vi "Marvin.vi"() -> ()   [LabVIEW 2017]
uses:
  Fuse_LW/Fuse25A_Labview/CANalystII/PCAN_Driver/ControlCAN.llb/CAN Channel.ctl
  CAN TxRx/CAN/CANalystII/PCAN_Driver/ControlCAN.llb/DevType.ctl
  CAN TxRx/CAN/CANalystII/PCAN_Driver/ControlCAN.llb/VCI_INIT_CONFIG.ctl
  CAN TxRx/CAN/CANalystII/PCAN_Driver/ControlCAN.llb/InitFlag.ctl
  CAN TxRx/CAN/CANalystII/PCAN_Driver/ControlCAN.llb/Fliter.ctl
  CAN TxRx/CAN/CANalystII/PCAN_Driver/ControlCAN.llb/Mode.ctl
  CAN TxRx/CAN/CANalystII/PCAN_Driver/ControlCAN.lvlib
panel:
  in  "lock":bool=TRUE
  in  "Display":bool
  in  "address":u16=341 format="%.0x"
  out "UnitType":T1(ring)
  in  "ch2_old":dbl
  in  "ch1_old":dbl
  out "ADC Units 6":dbl
  out "Config_CANAT":T8 {"DevType" items=["USB-CAN"=3, "USB-CAN2"=4]; "CanIndex" items=["通道1", "通道2"]; "VCI_INIT_CONFIG"."Fliter" items=["接收所有类型"=3, "只接收标准帧"=4, "只接收扩展帧"=7]; "VCI_INIT_CONFIG"."Mode" items=["正常工作", "自测模式（环回）", "仅侦听模式"]; "VCI_INIT_CONFIG"."InitFlag" items=["使用Flash参数", "使用界面设置参数"]}
  in  "Channel 2":T3 caption="Channel" items=["Channel 1", "Channel 2"]
  in  "CANType":u16(ring) items=["LAWICEL", "PCAN", "CANalystII"]
  out "error out 7":errorcluster
  out "error out 2":errorcluster
  in  "Clear History":bool
  in  "Time":i32=-1
  out "History":string
  in  "Tab Control":T9(tab)
  in  "Status 1":bool
  in  "Status":bool
  in  "SN":string
  in  "Get Version":bool
  out "Unit PN":string
  out "SW ver":string
  in  "Get SN":bool
  in  "Set SN":bool
  in  "Get PN":bool
  in  "Clear Time Log":bool
  in  "Clear Log":bool
  out "Event Logs":string
  in  "Clear Event Logs":bool
  in  "TxID":u32 format="%.0x"
  in  "Data":u8[](array[numeric])
  in  "Sent Debug":bool
  in  "Unit SN":bool
  in  "Bootloader":bool
  in  "Ethernet Config. Data":string
  in  "SendData":bool
  in  "ReadParam":bool
  in  "Unit reset":bool
  in  "SW ver":bool
  in  "MAC address":bool
  out "RX Cnt":u32
  out "TX Cnt":u32
  in  "stop m":bool
  out "error out 5":errorcluster
  out "error out 6":errorcluster
  out "erroro5 2":errorcluster
  out "erroro5":errorcluster
  out "error out 4":errorcluster
  out "VISA res_out":refnum<visa-resource-name>
  in  "Seria- Port":refnum<visa-resource-name>="COM5"
  out "error out 3":errorcluster
  out "error02":errorcluster
  out "error out":errorcluster
  out "RX":bool
  out "TX":bool
  in  "Disonnect":bool
  in  "Connect":bool
  out "CommIcon":bool=TRUE
  in  "UIFlagStop":bool
  in  "RXFlagStop":bool
  in  "TXFlagStop":bool
  out "Error":string
  out "Adapter Version":string
  in  "Baud":u16(ring)=284 items=["1M"=20, "500K"=28, "250K"=284, "125K"=796, "100K"=17199, "50K"=18223, "20K"=21295, "10K"=26415, "5K"=32639]
  # "[msec]"
  # "Save Data"
  # "[sec]"
  # "[msec]"
  # "DO 3"
  # "DO 4"
  # "DO 5"
  # "DO 6"
  # "DO 7"
  # "DO 8"
  # "DO 9"
  # "DO 10"
  # "DO 11"
  # "DO 12"
  # "DO 13"
  # "DO 14"
  # "DO 15"
  # "DO 16"
  # "ver 1.0"
  # "Channel Parameter"
  # "** 0-Infinity"
  # "System Parameters"
  # "Digital input status"
  # "*255-Infinity"
  # "DI 17"
  # "DI 18"
  # "DI 19"
  # "**"
  # "DI 20"
  # "DI 21"
  # "DI 22"
  # "DI 23"
  # "DI 24"
  # "DI 25"
  # "*"
  # "DI 26"
  # "DI 27"
  # "DI 28"
  # "*65535-always On"
  # "*"
  # "*65535-OFF"
  # "OC command"
  # "OC1"
  # "BIT"
  # "Production Data"
  # "OC2"
  # "Unit S/N"
  # "Offset Data"
  # "Custom Message"
  # "Channel Data"
  # "Channel Protection"
  # "Marvin"
  # "REDLER TECHNOLOGIES LTD"
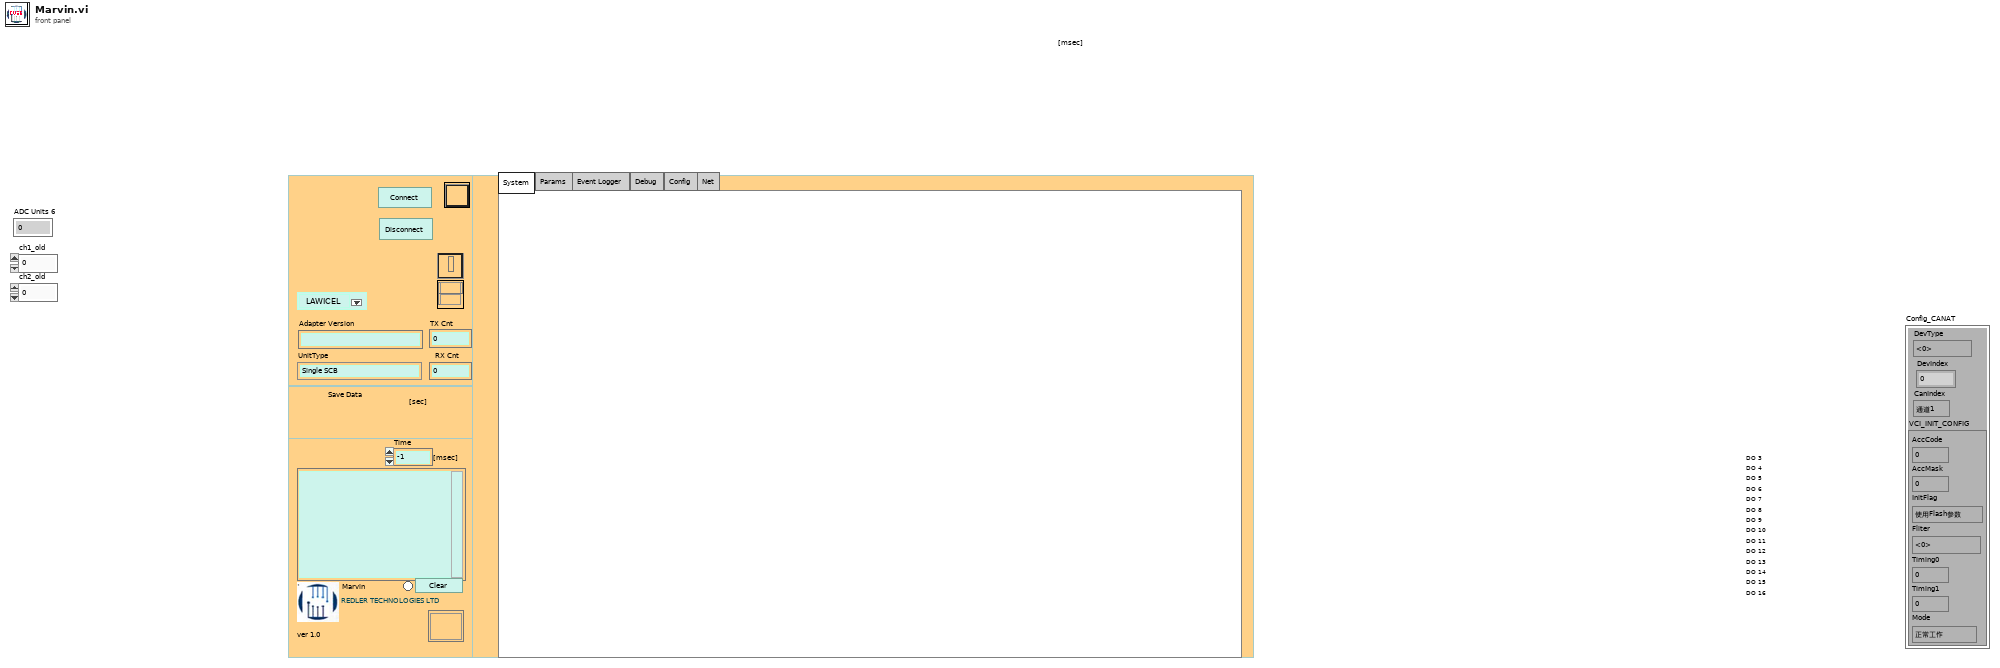
[diagram p1: front panel]
types:
  T1 = enum16{"Single SCB", "Power Rider", "Power Rider&Next10", "HATAL", "DAPH", "Indefinite", "Power Rider 12"}
  T2 = typedef "ControlCAN.lvlib/DevType.ctl" = u32
  T3 = typedef "ControlCAN.lvlib/CAN Channel.ctl" = u32
  T4 = typedef "ControlCAN.lvlib/VCI_INIT_CONFIG.ctl" = cluster{"AccCode":u32, "AccMask":u32, "InitFlag":T5, "Fliter":T6, "Timing0":u8, "Timing1":u8, "Mode":T7}
  T5 = typedef "ControlCAN.lvlib/InitFlag.ctl" = u32
  T6 = typedef "ControlCAN.lvlib/Fliter.ctl" = u8
  T7 = typedef "ControlCAN.lvlib/Mode.ctl" = u8
  T8 = cluster{"DevType":T2, "DevIndex":u32, "CanIndex":T3, "VCI_INIT_CONFIG":T4}
  T9 = enum32{"System", "Params", "Event Logger", "Debug", "Config", "Net"}
  T10 = enum16{"Single SCB", "Power Rider", "Power Rider&Next10", "HATAL", "DAPH", "Indefinite"}
  T11 = cluster{"ID":u32, "MSGTYPE":u8, "LEN":u8, "aDATA":u8[]}
  T12 = typedef "PCAN_ERROR.ctl" = i32
  T13 = cluster{"Is Warning":bool, "Is Error":bool, "Message":string}
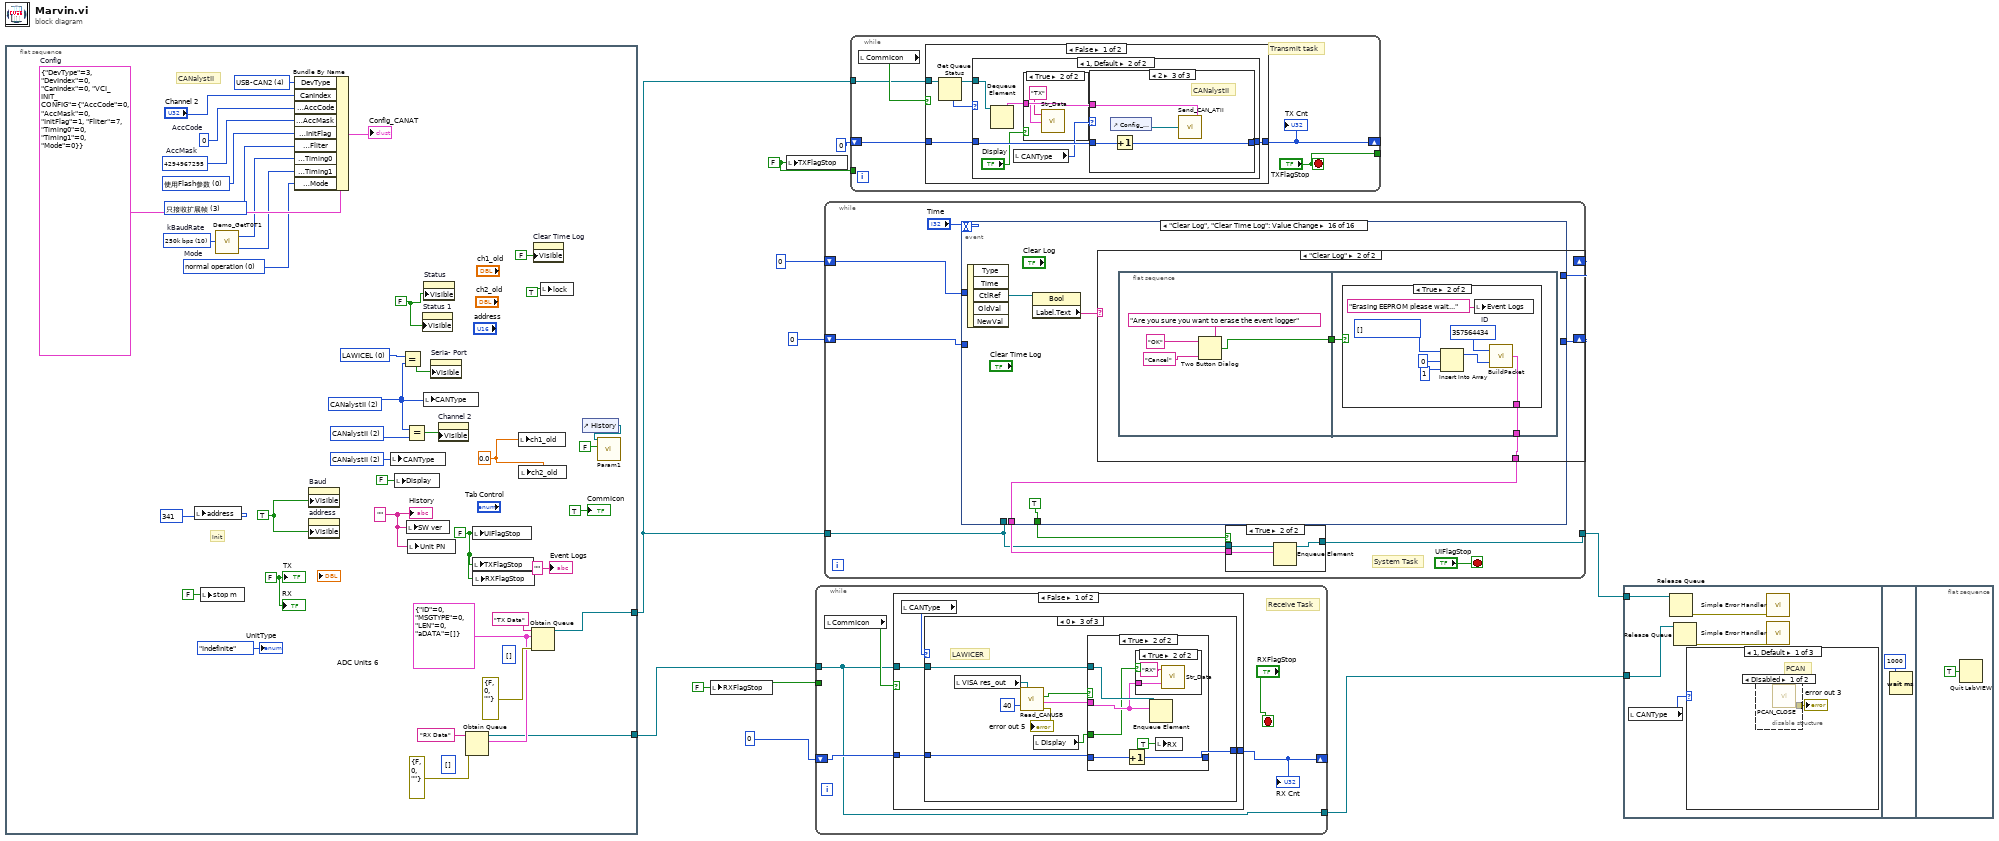
[diagram p0: block diagram]
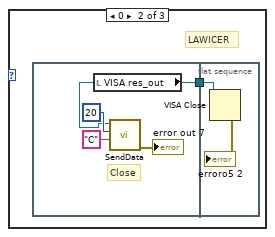
[diagram p3: hidden frame]
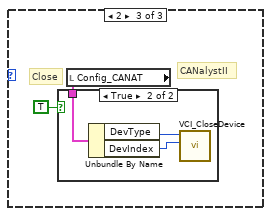
[diagram p4: hidden frame]
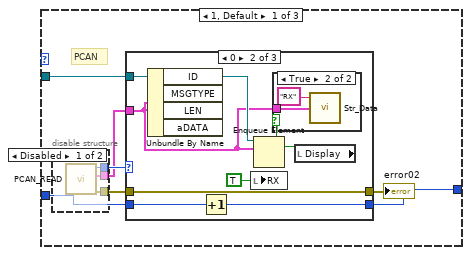
[diagram p6: hidden frame]
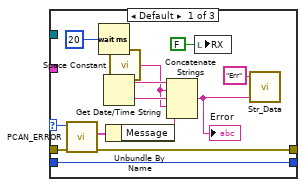
[diagram p8: hidden frame]
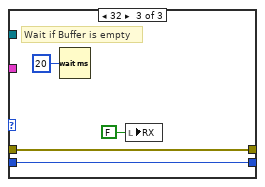
[diagram p10: hidden frame]
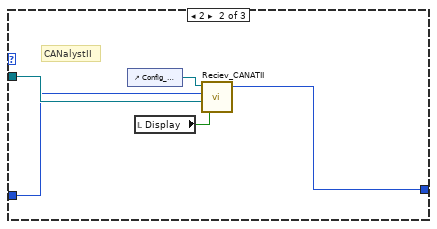
[diagram p11: hidden frame]
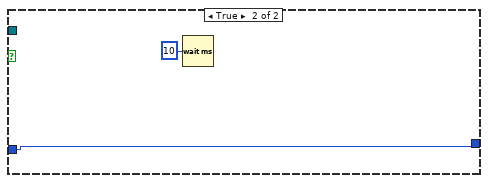
[diagram p14: hidden frame]
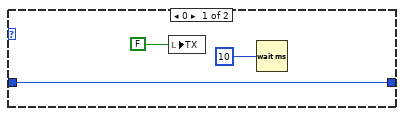
[diagram p15: hidden frame]
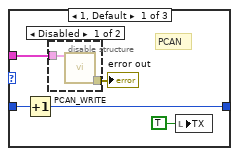
[diagram p17: hidden frame]
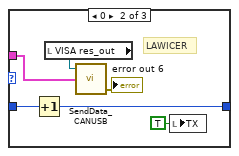
[diagram p19: hidden frame]
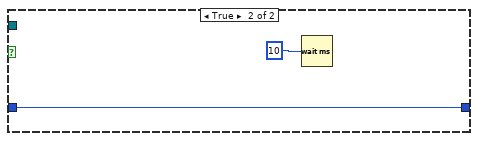
[diagram p20: hidden frame]
diagram:
  w4 = FALSE ("TXFlagStop")
  w5 = FALSE ("RXFlagStop")
  n1 = flat-sequence {
    tunnel: [w47] -> w8
    tunnel: [w45] -> w7
    frame #0 {
      w17 = "" ("str out")
      w19 = 0.0 ("ch1_old")
      w26 = TRUE ("Visible")
      w25 = u16 2 items=["LAWICEL", "PCAN", "CANalystII", "TCP Client", "TCP Server"] ("CANType")
      w23 = u16 2 items=["LAWICEL", "PCAN", "CANalystII", "TCP Client", "TCP Server"] ("CANType")
      w24 = u16 2 items=["LAWICEL", "PCAN", "CANalystII", "TCP Client", "TCP Server"] ("CANType")
      w22 = u16 0 items=["LAWICEL", "PCAN", "CANalystII", "TCP Client", "TCP Server"] ("CANType")
      w39 = u32 4294967295  # AccMask
      w38 = T5 0 items=["使用Flash参数", "使用界面设置参数"] ("InitFlag")
      w33 = T7 0 items=["normal operation", "Listen-only mode", "test mode"]  # Mode
      w37 = T6 3 items=["接收所有类型"=1, "只接收标准帧"=2, "只接收扩展帧"=3] ("Fliter")
      w36 = u8 10 items=["5k bps"=1, "10k bps"=2, "20k bps"=3, "40k bps"=4, "50k bps"=5, "80k bps"=6, "100k bps"=7, "125k bps"=8, "200k bps"=9, "250k bps"=10, "400k bps"=11, "500k bps"=12, "666k bps"=13, "800k bps"=14, "1000k bps"=15, "33.33k bps"=16, "66.66k bps"=17, "83.33k bps"=18]  # kBaudRate
      w40 = u32 0  # AccCode
      w42 = T2 4 items=["USB-CAN"=3, "USB-CAN2"=4] ("DevType")
      w43 = T8 {"DevType"=3, "DevIndex"=0, "CanIndex"=0, "VCI_INIT_CONFIG"={"AccCode"=0, "AccMask"=0, "InitFlag"=1, "Fliter"=7, "Timing0"=0, "Timing1"=0, "Mode"=0}}  # Config
      w31 = FALSE ("Visible")
      w27 = FALSE ("TX")
      w46 = T11 {"ID"=0, "MSGTYPE"=0, "LEN"=0, "aDATA"=[]} ("Msg")
      (unwired) u8[] []
      (unwired) u8[] []
      w11 = FALSE ("UIFlagStop")
      # "CANalystII"
      # "Init"
      n2 = local write "address"(u16 341 ("address-type")) -> ()
      n3 = local write "stop m"(FALSE ("stop m")) -> ()
      n4 = call "Demo_GetT0T1.vi"("kBaudRate"=w36) -> ("Timing0"=w35:u8, "Timing1"=w34:u8)
      n5 = Bundle By Name(cluster=w43, "DevType"=w42, "CanIndex"="Channel 2", "VCI_INIT_CONFIG.AccCode"=w40, "VCI_INIT_CONFIG.AccMask"=w39, "VCI_INIT_CONFIG.InitFlag"=w38, "VCI_INIT_CONFIG.Fliter"=w37, "VCI_INIT_CONFIG.Timing0"=w35, "VCI_INIT_CONFIG.Timing1"=w34, "VCI_INIT_CONFIG.Mode"=w33) -> (→"Config_CANAT":T8)
      n6 = property on="Baud" class="Ring (strict)"("Visible"=w26) -> ()  [unwired: 2 in, 2 out]
      n7 = property on="address" class="DigNum (strict)"("Visible"=w26) -> ()  [unwired: 2 in, 2 out]
      n8 = local write "CANType"(w25) -> ()
      n9 = local write "Display"(FALSE ("Display")) -> ()
      n10 = Equal?(x=w22, y=w24) -> (x = y?=w20:bool)
      n11 = Equal?(x=w24, y=w23) -> (x = y?=w21:bool)
      n12 = local write "SW ver"(w17) -> ()
      n13 = local write "Unit PN"(w17) -> ()
      n14 = property on="Status 1" class="Bool"("Visible"=w31) -> ()  [unwired: 2 in, 2 out]
      n15 = local write "CANType"(w24) -> ()
      n16 = property on="Status" class="Bool"("Visible"=w31) -> ()  [unwired: 2 in, 2 out]
      n17 = property on="Seria- Port" class="VISAName"("Visible"=w20) -> ()  [unwired: 2 in, 2 out]
      n18 = property on="Channel 2" class="Ring (strict)"("Visible"=w21) -> ()  [unwired: 2 in, 2 out]
      n19 = Obtain Queue(name (unnamed)="RX Data", element data type=w46, error in (no error)=errorcluster {"status"=FALSE, "code"=0, "source"=""}) -> (queue out=w45:refnum<queue>)  [unwired: 2 in, 2 out]
      n20 = local write "UIFlagStop"(w11) -> ()
      n21 = local write "TXFlagStop"(w11) -> ()
      n22 = local write "RXFlagStop"(w11) -> ()
      n23 = local write "ch1_old"(w19) -> ()
      n24 = local write "ch2_old"(w19) -> ()
      n25 = Obtain Queue(name (unnamed)="TX Data", element data type=w46, error in (no error)=errorcluster {"status"=FALSE, "code"=0, "source"=""}) -> (queue out=w47:refnum<queue>)  [unwired: 2 in, 2 out]
      n26 = property on="Clear Time Log" class="Bool"("Visible"=FALSE) -> ()  [unwired: 2 in, 2 out]
      n27 = local write "lock"(TRUE ("lock")) -> ()
      n28 = control-ref of="History"() -> (w16:refnum<vi>)
      n29 = call "Param1.vi"("str"=w16, "Init_F"=FALSE) -> ()  [unwired: 16 in, 2 out]
      "RX" <- w27
      "TX" <- w27
      "Event Logs" <- "" ("Event Logs")
      "UnitType" <- T10."Indefinite" ("UnitType")
      "CommIcon" <- TRUE ("CommIcon")
      "History" <- w17
    }
  }
  n30 = local write "RXFlagStop"(w5) -> ()
  n31 = local write "TXFlagStop"(w4) -> ()
  n32 = while {
    tunnel: w7 -> [w52]
    shift-right: [w53] -> _
    shift-left: u32 0 ("cnt_out") -> [w54]
    tunnel: w5 -> [_]
    tunnel: [w52] -> w2
    stop <- "RXFlagStop" stop-if-true
    # "Receive Task"
    n33 = local read "CommIcon"() -> (w55:bool)
    n34 = case shown="False" w55 {
      tunnel: w52 -> [w60 _]
      tunnel: w54 -> [w58 w120]
      tunnel: [w57 w120] -> w53
      frame False {
        n35 = local read "CANType"() -> (w59:u16)
        n36 = case shown="0" w59 {
          tunnel: w60 -> [w64 w100 w107]
          tunnel: w58 -> [w62 w99 w104]
          tunnel: [w61 w98 w103] -> w57
          frame 1, Default {
            # "PCAN"
            n37 = disable-structure shown="Disabled" {
              disable-tunnel: [w70 _] -> w67
              disable-tunnel: [w69 _] -> w66
              disable-tunnel: [w68 _] -> w65
              frame Disabled {
                n38 = call "PCAN_READ.vi"() -> ("error out"=w70:errorcluster, "TPCANMsg"=w68:T11, "error"=w69:T12)  [unwired: 2 in, 7 out]
              }
              frame Enabled {
              }
            }
            n39 = case shown="0" w66 {
              selector: w66 -> [w82 _ _]
              tunnel: w65 -> [_ w86 _]
              tunnel: w67 -> [w83 w90 w95]
              tunnel: [w81 w90 w95] -> w63
              tunnel: w64 -> [_ w89 _]
              tunnel: w62 -> [w73 w85 w93]
              tunnel: [w73 w87 w93] -> w61
              frame Default {
                n40 = call "PCAN_ERROR.vi"("error in (no error)"=w83, "Error Code"=w82) -> ("error out"=w81:errorcluster, "PCAN error"=w80:T13)  [unwired: 8 out]
                n41 = Wait (ms)(milliseconds to wait=u32 20) -> ()  [unwired: 1 out]
                n42 = Get Date/Time String() -> (date string=w78:string, time string=w77:string)  [unwired: 3 out]
                n43 = Unbundle By Name(w80) -> ("Message"=w76:string)
                n44 = call <vilib>:"Space Constant.vi"() -> ("String"=w75:string)
                n45 = Concatenate Strings(w78, w75, w77, w75, w76) -> (w71:string)
                "Error" <- w71
                n46 = local write "RX"(FALSE ("RX")) -> ()
                n47 = call "Str_Data.vi"("Err str"=w71, "string"="Err") -> ()  [unwired: 1 in, 1 out]
              }
              frame 0 {
                n48 = Unbundle By Name(w86) -> ()  [unwired: 4 out]
                n49 = Increment(x=w85) -> (x+1=w87:u32)
                n50 = local write "RX"(TRUE ("RX")) -> ()
                n51 = Enqueue Element(queue=w89, element=w86) -> ()  [unwired: 1 in, 4 out]
                n52 = local read "Display"() -> (w84:bool)
                n53 = case shown="True" w84 {
                  tunnel: w86 -> [_ w91]
                  frame False {
                  }
                  frame True {
                    n54 = call "Str_Data.vi"("Msg"=w91, "string"="RX") -> ()  [unwired: 1 in, 1 out]
                  }
                }
              }
              frame 32 {
                # "Wait if Buffer is empty"
                n55 = Wait (ms)(milliseconds to wait=u32 20) -> ()  [unwired: 1 out]
                n56 = local write "RX"(FALSE ("RX")) -> ()
              }
            }
            "error02" <- w63
          }
          frame 2 {
            # "CANalystII"
            n57 = control-ref of="Config_CANAT"() -> (w101:refnum<vi>)
            n58 = local read "Display"() -> (w97:bool)
            n59 = call "Reciev_CANATII.vi"("Display"=w97, "queue out"=w100, "cnd_in"=w99, "Config"=w101) -> ("cnt_out"=w98:u32)  [unwired: 2 out]
          }
          frame 0 {
            # "LAWICER"
            n60 = local read "VISA res_out"() -> (w110:refnum<visa-resource-name>)
            n61 = call "Read_CANUSB.vi"("VISA  in"=w110, "byte count"=u32 40) -> ("Status"=w105:bool, "TPCANMsg out"=w106:T11, "error out 5"=→"error out 5":errorcluster)  [unwired: 2 out]
            n62 = local read "Display"() -> (w102:bool)
            n63 = case shown="True" w105 {
              tunnel: w107 -> [_ w116]
              tunnel: w106 -> [_ w113]
              tunnel: w104 -> [w111 w115]
              tunnel: [w111 w114] -> w103
              tunnel: w102 -> [_ w112]
              frame False {
              }
              frame True {
                n64 = Increment(x=w115) -> (x+1=w114:u32)
                n65 = case shown="True" w112 {
                  tunnel: w113 -> [_ w118]
                  frame False {
                  }
                  frame True {
                    n66 = call "Str_Data.vi"("Msg"=w118, "string"="RX") -> ()  [unwired: 1 in, 1 out]
                  }
                }
                n67 = Enqueue Element(queue=w116, element=w113) -> ()  [unwired: 1 in, 4 out]
                n68 = local write "RX"(TRUE ("RX")) -> ()
              }
            }
          }
        }
      }
      frame True {
        n69 = Wait (ms)(milliseconds to wait=u32 10) -> ()  [unwired: 1 out]
      }
    }
    "RX Cnt" <- w53
  }
  n70 = while {
    tunnel: w8 -> [w128]
    tunnel: [w127] -> w1
    shift-right: [w125] -> _
    shift-left: u32 0 -> [w126]
    shift-right: [w123] -> _
    shift-left: u32 0 -> [w124]
    stop <- "UIFlagStop" stop-if-true
    # "System Task"
    n71 = event shown="[15] \"Clear Log\", \"Clear Time Log\": Value Change" {
      selector: _ -> [_ _ _ _ _ _ _ _ _ _ _ _ _ _ _ _]
      dyn-events: _ -> [_ _ _ _ _ _ _ _ _ _ _ _ _ _ _ _]
      timeout: "Time" -> [_ _ _ _ _ _ _ _ _ _ _ _ _ _ _ _]
      tunnel: [_ w141 _ w164 _ w206 w212 w218 _ _ w251 w253 _ _ _ w283] -> w131
      tunnel: [_ TRUE ("TX") FALSE ("TX") w165 FALSE TRUE TRUE TRUE FALSE FALSE TRUE _ FALSE FALSE _ TRUE] -> w130
      tunnel: w126 -> [_ _ w159 _ _ _ _ _ _ w237 _ _ _ _ _ _]
      tunnel: [_ _ w159 _ _ _ _ _ _ w237 _ _ _ _ _ _] -> w125
      tunnel: w128 -> [_ _ _ _ _ _ _ _ _ _ _ _ _ _ _ _]
      tunnel: w124 -> [_ _ w160 _ _ _ w208 w214 w220 _ w248 _ _ _ _ _]
      tunnel: [_ _ w160 _ _ _ w208 w214 w220 _ w248 _ _ _ _ _] -> w123
      event Timeout {
        n72 = event-data() -> ()  [unwired: 1 in, 1 out]
      }
      event "SendData", "ReadParam", "Unit reset", "SW ver", "Bootloader", "Unit SN", "MAC address": Value Change {
        w146 = u8 2 items=["STATUS"=128, "EXTENDED"=2, "RTR"=1, "DATA MSG"=0] ("MSGTYPE")
        n73 = event-data() -> ("CtlRef"=w139:refnum<vi>)  [unwired: 1 in]
        n74 = property class="Bool"(reference=w139) -> ("Label.Text"=w138:string)  [unwired: 1 in, 2 out]
        n75 = case shown="\"SendData\"" w138 {
          tunnel: ["" ("Ethernet Configuration Data") "Ethernet Config. Data" "netparam" ("Ethernet Configuration Data") "reset" ("Ethernet Configuration Data") "version" ("Ethernet Configuration Data") "boot" ("Ethernet Configuration Data") "serial" ("Ethernet Configuration Data") "mac" ("Ethernet Configuration Data")] -> w137
          frame "False", Default {
          }
          frame "SendData" {
          }
          frame "ReadParam" {
            # "read param."
          }
          frame "Unit reset" {
            # "reset"
          }
          frame "SW ver" {
            # "sw ver"
          }
          frame "Bootloader" {
            # "Bootloader"
          }
          frame "Unit SN" {
            # "S/N"
          }
          frame "MAC address" {
            # "MAC"
          }
        }
        n76 = String To Byte Array(string=w137) -> (unsigned byte array=w136:u8[])
        n77 = Array Size(array=w136) -> (size(s)=w143:i32)
        n78 = To Unsigned Byte Integer(number=w143) -> (unsigned 8bit integer=w145:u8)
        n79 = Bundle By Name(cluster=T11 {"ID"=0, "MSGTYPE"=0, "LEN"=0, "aDATA"=[]} ("MsgTX 2"), "ID"=u32 0, "MSGTYPE"=w146, "LEN"=w145, "aDATA"=w136) -> (w141:T11)
      }
      event "lock": Value Change {
        n80 = event-data() -> ()  [unwired: 1 in, 1 out]
        n81 = call "EnterPW.vi"() -> ("Prod"=w155:bool, "Tech"=w158:bool)  [unwired: 7 in, 2 out]
        n82 = Or(x=w158, y=w155) -> (x .or. y?=w157:bool)
        n83 = Not(x=w157) -> (.not. x?=w156:bool)
        n84 = call "PWVisibleCntl.vi"("Tech"=w158, "Product"=w155) -> ()  [unwired: 14 in]
        n85 = local write "lock"(w156) -> ()
        n86 = property on="Clear Time Log" class="Bool"("Visible"=w155) -> ()  [unwired: 2 in, 2 out]
      }
      event "Connect": Value Change {
        w167 = 0 items=["extended", "standart"] ("type")
        n87 = event-data() -> ()  [unwired: 1 in, 1 out]
        n88 = case shown="2" "CANType" {
          tunnel: [w178 w186 w197] -> w163
          tunnel: [w180 "CANalystII" ("read ver") w198] -> w166
          tunnel: "Baud" -> [w177 w189 w196]
          tunnel: w167 -> [w176 w188 _]
          frame 1, Default {
            # "PCAN"
            n89 = disable-structure shown="Disabled" {
              disable-tunnel: [w184 _] -> w180
              disable-tunnel: [w183 _] -> w179
              disable-tunnel: w177 -> [w182 _]
              disable-tunnel: w176 -> [w181 _]
              frame Disabled {
                n90 = call "Init_PCAN.vi"("type"=w181, "baud"=w182) -> ("Boolean"=w183:bool, "Version"=w184:string)
              }
              frame Enabled {
              }
            }
            n91 = Not(x=w179) -> (.not. x?=w178:bool)
          }
          frame 2 {
            # "CANalystII"
            n92 = flat-sequence {
              tunnel: w189 -> [w192]
              tunnel: w188 -> [_]
              tunnel: [w191] -> w185
              tunnel: [w194] -> w187
              tunnel: w185 -> [w193]
              frame #0 {
                n93 = control-ref of="Config_CANAT"() -> (w191:refnum<vi>)
                n94 = call "ChangeCANBaud.vi"("baud in"=w192, "reference"=w191) -> ()
              }
              frame #1 {
                n95 = call "InitCAN_ATII.vi"("Config"=w193) -> ("Sts"=w194:bool)
              }
            }
            n96 = Not(x=w187) -> (.not. x?=w186:bool)
          }
          frame 0 {
            # "LAWICER"
            n97 = call "Init_Lawicel.vi"("baud"=w196, "Seria- Port"="Seria- Port") -> ("error out 4"=→"error out 4":errorcluster, "Status"=w195:bool, "read ver"=w198:string, "VISA res_out"=→"VISA res_out":refnum<visa-resource-name>)  [unwired: 1 in]
            n98 = Not(x=w195) -> (.not. x?=w197:bool)
          }
        }
        "Adapter Version" <- w166
        n99 = Not(x=w163) -> (.not. x?=w162:bool)
        n100 = case shown="True" w162 {
          tunnel: [FALSE TRUE] -> w165
          tunnel: [T11 {"ID"=0, "MSGTYPE"=0, "LEN"=0, "aDATA"=[]} ("MsgTX 2") w172] -> w164
          frame False {
          }
          frame True {
            w174 = u32 357564455  # ID
            # "PN"
            # "0x15500027"
            n101 = call "BuildPacket.vi"("Data"=u8[] [] ("Data 2"), "TxID"=w174) -> ("MsgTX 2"=w172:T11)
          }
        }
        n102 = local write "CommIcon"(w163) -> ()
      }
      event "stop m": Value Change {
        w202 = TRUE ("UIFlagStop")
        n103 = event-data() -> ()  [unwired: 1 in, 1 out]
        n104 = local write "UIFlagStop"(w202) -> ()
        n105 = local write "TXFlagStop"(w202) -> ()
        n106 = local write "RXFlagStop"(w202) -> ()
      }
      event "Sent Debug": Value Change {
        n107 = event-data() -> ()  [unwired: 1 in, 1 out]
        n108 = call "BuildPacket.vi"("Data"="Data", "TxID"="TxID") -> ("MsgTX 2"=w206:T11)
      }
      event "Get Version": Value Change {
        w210 = u32 357564425  # ID
        # "Version"
        # "0x15500009"
        n109 = event-data() -> ()  [unwired: 1 in, 1 out]
        n110 = call "BuildPacket.vi"("Data"=u8[] [] ("Data 2"), "TxID"=w210) -> ("MsgTX 2"=w212:T11)
        "SW ver" <- "" ("SW ver")
      }
      event "Get PN": Value Change {
        w216 = u32 357564455  # ID
        # "P/N"
        # "0x15500027"
        n111 = event-data() -> ()  [unwired: 1 in, 1 out]
        n112 = call "BuildPacket.vi"("Data"=u8[] [] ("Data 2"), "TxID"=w216) -> ("MsgTX 2"=w218:T11)
        "Unit PN" <- "" ("SW ver")
      }
      event "Get SN", "Set SN": Value Change {
        # "SN"
        n113 = event-data() -> ("CtlRef"=w222:refnum<vi>)  [unwired: 1 in]
        n114 = property class="Bool"(reference=w222) -> ("Label.Text"=w221:string)  [unwired: 1 in, 2 out]
        n115 = case shown="\"Get SN\", Default" w221 {
          frame "Get SN", Default {
            n116 = call "SN_Data.vi"("type"=1) -> ()  [unwired: 10 in, 1 out]
            n117 = local write "SN"("" ("SN")) -> ()
          }
          frame "Set SN" {
            n118 = call "SN_Data.vi"("type"=0, "String"="SN") -> ()  [unwired: 9 in, 1 out]
          }
        }
      }
      event "CANType": Value Change {
        w234 = u16 2 items=["LAWICEL", "PCAN", "CANalystII"] ("CANType")
        w235 = u16 0 items=["LAWICEL", "PCAN", "CANalystII"] ("CANType")
        n119 = event-data() -> ()  [unwired: 1 in, 1 out]
        n120 = local read "CANType"() -> (w231:u16)
        n121 = case shown="1" w231 {
          tunnel: [w241 w244 w247] -> w230
          tunnel: [w241 w244 w247] -> w229
          tunnel: [FALSE ("TX") FALSE ("TX") FALSE ("TX")] -> _
          tunnel: [FALSE ("TX") FALSE ("TX") FALSE ("TX")] -> w228
          frame 0, Default {
            w241 = TRUE ("TX")
            # "Lawicel"
          }
          frame 1 {
            w244 = TRUE ("TX")
            # "PCAN"
          }
          frame 2 {
            w247 = TRUE ("TX")
            # "CANalystll"
          }
        }
        n122 = property on="Connect" class="Bool"("Visible"=w229) -> ()  [unwired: 2 in, 2 out]
        n123 = property on="Disonnect" class="Bool"("Visible"=w229) -> ()  [unwired: 2 in, 2 out]
        n124 = property on="Baud" class="Ring (strict)"("Visible"=w230) -> ()  [unwired: 2 in, 2 out]
        n125 = property on="address" class="DigNum (strict)"("Visible"=w230) -> ()  [unwired: 2 in, 2 out]
        n126 = local read "CANType"() -> (w232:u16)
        n127 = Equal?(x=w235, y=w232) -> (x = y?=w236:bool)
        n128 = Equal?(x=w232, y=w234) -> (x = y?=w233:bool)
        n129 = local write "CANType"(w232) -> ()
        n130 = property on="Channel 2" class="Ring (strict)"("Visible"=w233) -> ()  [unwired: 2 in, 2 out]
        n131 = property on="Seria- Port" class="VISAName"("Visible"=w236) -> ()  [unwired: 2 in, 2 out]
        n132 = property on="SendData" class="Bool"("Visible"=w228) -> ()  [unwired: 2 in, 2 out]
        n133 = property on="ReadParam" class="Bool"("Visible"=w228) -> ()  [unwired: 2 in, 2 out]
        n134 = property on="Unit reset" class="Bool"("Visible"=w228) -> ()  [unwired: 2 in, 2 out]
        n135 = property on="SW ver" class="Bool"("Visible"=w228) -> ()  [unwired: 2 in, 2 out]
        n136 = property on="Unit SN" class="Bool"("Visible"=w228) -> ()  [unwired: 2 in, 2 out]
        n137 = property on="Bootloader" class="Bool"("Visible"=w228) -> ()  [unwired: 2 in, 2 out]
        n138 = property on="MAC address" class="Bool"("Visible"=w228) -> ()  [unwired: 2 in, 2 out]
      }
      event "Status": Value Change {
        w249 = u32 357564416  # ID
        # "Status"
        # "0x1550000"
        n139 = event-data() -> ()  [unwired: 1 in, 1 out]
        n140 = call "BuildPacket.vi"("Data"=u8[] [] ("Data 2"), "TxID"=w249) -> ("MsgTX 2"=w251:T11)
      }
      event "Status 1": Value Change {
        w254 = u32 357564417  # ID
        # "Status1"
        # "0x15500001"
        n141 = event-data() -> ()  [unwired: 1 in, 1 out]
        n142 = call "BuildPacket.vi"("Data"=u8[] [] ("Data 2"), "TxID"=w254) -> ("MsgTX 2"=w253:T11)
      }
      event "Disonnect": Value Change {
        # "Disconnect"
        n143 = event-data() -> ()  [unwired: 1 in, 1 out]
        n144 = local read "CANType"() -> (w257:u16)
        n145 = case shown="0" w257 {
          tunnel: [TRUE TRUE TRUE] -> w256
          frame 1, Default {
            # "PCAN"
            n146 = disable-structure shown="Disabled" {
              frame Disabled {
                n147 = call "PCAN_CLOSE.vi"() -> ()  [unwired: 1 in, 11 out]
              }
              frame Enabled {
              }
            }
            n148 = local write "UnitType"(T10."Indefinite" ("UnitType")) -> ()
          }
          frame 2 {
            # "CANalystII"
            # "Close"
            n149 = local read "Config_CANAT"() -> (w263:T8)
            n150 = case shown="True" TRUE {
              tunnel: w263 -> [_ w267]
              frame False {
              }
              frame True {
                n151 = Unbundle By Name(w267) -> ("DevType"=w266:T2, "DevIndex"=w265:u32)
                n152 = call "VCI_CloseDevice.vi"("DevIndex"=w265, "DevType"=w266) -> ()  [unwired: 1 in, 9 out]
              }
            }
            n153 = local write "UnitType"(T10."Indefinite" ("UnitType")) -> ()
          }
          frame 0 {
            # "LAWICER"
            n154 = flat-sequence {
              tunnel: [w272] -> w269
              tunnel: w269 -> [w276]
              frame #0 {
                # "Close"
                n155 = local read "VISA res_out"() -> (w272:refnum<visa-resource-name>)
                n156 = call "SendData.vi"("String"="C", "byte count"=u32 20, "VISA resource name out 2"=w272) -> ("error out"=→"error out 2":errorcluster)  [unwired: 1 in, 3 out]
              }
              frame #1 {
                n157 = VISA Close(VISA resource name=w276) -> (error out=→"erroro5":errorcluster)  [unwired: 1 in]
              }
            }
            n158 = local write "UnitType"(T10."Indefinite" ("UnitType")) -> ()
          }
        }
        n159 = local write "CommIcon"(w256) -> ()
      }
      event "Clear History": Value Change {
        n160 = event-data() -> ()  [unwired: 1 in, 1 out]
        n161 = local write "History"("" ("str out")) -> ()
      }
      event "Clear Event Logs": Value Change {
        n162 = event-data() -> ()  [unwired: 1 in, 5 out]
        n163 = local write "Event Logs"("" ("Event Logs")) -> ()
      }
      event "Clear Log", "Clear Time Log": Value Change {
        n164 = event-data() -> ("CtlRef"=w281:refnum<vi>)  [unwired: 1 in, 4 out]
        n165 = property class="Bool"(reference=w281) -> ("Label.Text"=w280:string)  [unwired: 1 in, 2 out]
        n166 = case shown="\"Clear Log\"" w280 {
          tunnel: [w284 w299] -> w283
          frame "Clear Time Log", Default {
            n167 = flat-sequence {
              tunnel: [w286] -> w285
              tunnel: [w291] -> w284
              tunnel: w285 -> [w290]
              frame #0 {
                n168 = Two Button Dialog(message="Are you sure you want to reset the system time", 1:"Cancel" ("F button name (\"Cancel\")"), 2:"OK" ("T button name (\"OK\")")) -> (T button?=w286:bool)
              }
              frame #1 {
                n169 = case shown="True" w290 {
                  tunnel: [_ w294] -> w291
                  frame False {
                  }
                  frame True {
                    w298 = u32 357564434  # ID
                    n170 = Insert Into Array(array=u8[] [] ("Data 2"), index=0, new element=u8 2 ("new element/subarray")) -> (w295:u8[])
                    n171 = local write "Event Logs"("System time reset" ("Event Logs")) -> ()
                    n172 = call "BuildPacket.vi"("Data"=w295, "TxID"=w298) -> ("MsgTX 2"=w294:T11)
                  }
                }
              }
            }
          }
          frame "Clear Log" {
            n173 = flat-sequence {
              tunnel: [w301] -> w300
              tunnel: [w306] -> w299
              tunnel: w300 -> [w305]
              frame #0 {
                n174 = Two Button Dialog(message="Are you sure you want to erase the event logger", 1:"Cancel" ("F button name (\"Cancel\")"), 2:"OK" ("T button name (\"OK\")")) -> (T button?=w301:bool)
              }
              frame #1 {
                n175 = case shown="True" w305 {
                  tunnel: [_ w309] -> w306
                  frame False {
                  }
                  frame True {
                    w313 = u32 357564434  # ID
                    n176 = Insert Into Array(array=u8[] [] ("Data 2"), index=0, new element=u8 1 ("new element/subarray")) -> (w310:u8[])
                    n177 = local write "Event Logs"("Erasing EEPROM please wait..." ("Event Logs")) -> ()
                    n178 = call "BuildPacket.vi"("Data"=w310, "TxID"=w313) -> ("MsgTX 2"=w309:T11)
                  }
                }
              }
            }
          }
        }
      }
    }
    n179 = case shown="True" w130 {
      tunnel: w128 -> [w132 w135]
      tunnel: [w132 w134] -> w127
      tunnel: w131 -> [_ w133]
      frame False {
      }
      frame True {
        n180 = Enqueue Element(queue=w135, element=w133) -> (queue out=w134:refnum<queue>)  [unwired: 1 in, 3 out]
      }
    }
  }
  n181 = while {
    tunnel: ["TXFlagStop"] -> _
    tunnel: w8 -> [w316]
    shift-right: [w314] -> _
    shift-left: u32 0 -> [w315]
    tunnel: w4 -> [_]
    stop <- "TXFlagStop" stop-if-true
    # "Transmit task"
    n182 = local read "CommIcon"() -> (w317:bool)
    n183 = case shown="False" w317 {
      tunnel: w316 -> [w323 _]
      tunnel: w315 -> [w320 w352]
      tunnel: [w319 w352] -> w314
      frame False {
        n184 = Get Queue Status(queue=w323) -> (queue out=w321:refnum<queue>, # elements in queue=w322:i32)  [unwired: 1 in, 7 out]
        n185 = case shown="1, Default" w322 {
          tunnel: w321 -> [_ w332]
          tunnel: w320 -> [w324 w331]
          tunnel: [w324 w330] -> w319
          frame 0 {
            n186 = local write "TX"(FALSE ("TX")) -> ()
            n187 = Wait (ms)(milliseconds to wait=u32 10) -> ()  [unwired: 1 out]
          }
          frame 1, Default {
            n188 = Dequeue Element(queue=w332) -> (element=w329:T11)  [unwired: 1 in, 4 out]
            n189 = local read "CANType"() -> (w328:u16)
            n190 = case shown="True" "Display" {
              tunnel: w329 -> [_ w333]
              frame False {
              }
              frame True {
                n191 = call "Str_Data.vi"("Msg"=w333, "string"="TX") -> ()  [unwired: 1 in, 1 out]
              }
            }
            n192 = case shown="2" w328 {
              tunnel: w329 -> [w339 w346 w348]
              tunnel: w331 -> [w336 w343 w351]
              tunnel: [w335 w342 w350] -> w330
              frame 1, Default {
                # "PCAN"
                n193 = Increment(x=w336) -> (x+1=w335:u32)
                n194 = disable-structure shown="Disabled" {
                  disable-tunnel: w339 -> [w341 _]
                  disable-tunnel: [w340 _] -> w338
                  frame Disabled {
                    n195 = call "PCAN_WRITE.vi"("TPCANMsg"=w341) -> ("error out"=w340:errorcluster)  [unwired: 2 in, 8 out]
                  }
                  frame Enabled {
                  }
                }
                "error out" <- w338
                n196 = local write "TX"(TRUE ("TX")) -> ()
              }
              frame 0 {
                # "LAWICER"
                n197 = Increment(x=w343) -> (x+1=w342:u32)
                n198 = local read "VISA res_out"() -> (w345:refnum<visa-resource-name>)
                n199 = call "SendData_CANUSB.vi"("Msg"=w346, "VISA res_in"=w345) -> ("error out 6"=→"error out 6":errorcluster)  [unwired: 1 in, 2 out]
                n200 = local write "TX"(TRUE ("TX")) -> ()
              }
              frame 2 {
                # "CANalystII"
                n201 = control-ref of="Config_CANAT"() -> (w349:refnum<vi>)
                n202 = Increment(x=w351) -> (x+1=w350:u32)
                n203 = call "Send_CAN_ATII.vi"("MsgTX"=w348, "Config"=w349) -> ()
              }
            }
          }
        }
      }
      frame True {
        n204 = Wait (ms)(milliseconds to wait=u32 10) -> ()  [unwired: 1 out]
      }
    }
    "TX Cnt" <- w314
  }
  n205 = flat-sequence {
    tunnel: w1 -> [w358]
    tunnel: w2 -> [w355]
    frame #0 {
      n206 = local read "CANType"() -> (w354:u16)
      n207 = Release Queue(queue=w358) -> (error out=w357:errorcluster)  [unwired: 1 in, 3 out]
      n208 = Release Queue(queue=w355) -> (error out=w356:errorcluster)  [unwired: 1 in, 3 out]
      n209 = case shown="1, Default" w354 {
        frame 1, Default {
          # "PCAN"
          n210 = disable-structure shown="Disabled" {
            disable-tunnel: [w360 _] -> w359
            frame Disabled {
              n211 = call "PCAN_CLOSE.vi"() -> ("error out"=w360:errorcluster)  [unwired: 1 in, 10 out]
            }
            frame Enabled {
            }
          }
          "error out 3" <- w359
        }
        frame 0 {
          # "LAWICER"
          n212 = flat-sequence {
            tunnel: [w363] -> w361
            tunnel: w361 -> [w367]
            frame #0 {
              # "Close"
              n213 = local read "VISA res_out"() -> (w363:refnum<visa-resource-name>)
              n214 = call "SendData.vi"("String"="C", "byte count"=u32 20, "VISA resource name out 2"=w363) -> ("error out"=→"error out 7":errorcluster)  [unwired: 1 in, 3 out]
            }
            frame #1 {
              n215 = VISA Close(VISA resource name=w367) -> (error out=→"erroro5 2":errorcluster)  [unwired: 1 in]
            }
          }
        }
        frame 2 {
          # "CANalystII"
          # "Close"
          n216 = local read "Config_CANAT"() -> (w369:T8)
          n217 = case shown="True" TRUE {
            tunnel: w369 -> [_ w370]
            frame False {
            }
            frame True {
              n218 = Unbundle By Name(w370) -> ("DevType"=w372:T2, "DevIndex"=w371:u32)
              n219 = call "VCI_CloseDevice.vi"("DevIndex"=w371, "DevType"=w372) -> ()  [unwired: 1 in, 9 out]
            }
          }
        }
      }
      n220 = call <vilib>:"Simple Error Handler.vi"("error in (no error)"=w357) -> ()  [unwired: 1 in, 8 out]
      n221 = call <vilib>:"Simple Error Handler.vi"("error in (no error)"=w356) -> ()  [unwired: 1 in, 8 out]
    }
    frame #1 {
      n222 = Wait (ms)(milliseconds to wait=u32 1000) -> ()  [unwired: 1 out]
    }
    frame #2 {
      n223 = Quit LabVIEW(quit? (T)=TRUE) -> ()
    }
  }
